vi "realtimecurrent.vi"() -> ()   [LabVIEW 2016]
uses:
  <vilib>/rvi/interface/nirviReadWriteControl/nirviReadWriteControl.xnode
  <vilib>/rvi/interface/nirviCloseFPGA/nirviCloseFPGA.xnode
  <vilib>/functionblocks/FB Core/FB Core.xnode
  <vilib>/rvi/interface/nirviOpenFPGA/nirviOpenFPGA.xnode
  <vilib>/userdefined/High Color/nirio_resource_hc.ctl
  NiFpgaLv.dll
  <vilib>/Utility/error.llb/Error Cluster From Error Code.vi
  <vilib>/rvi/errors/niLvFpgaAdjustHostInterfaceError.vi
  fpga/InjFPGA.vi
  <vilib>/functionblocks/Control/PID/PID.vi
  <vilib>/functionblocks/NI_FunctionBlock Libraries.lvlib
  FPGA Bitfiles/Controlsoftware2_FPGATarget_InjFPGA_-aTnSXeY2bA.lvbitx
  <vilib>/FPGAPlugInAG/cRIO-9074/niLvFpga_Open_cRIO-9074.vi
  <vilib>/FPGAPlugInAG/cRIO-9074/niLvFpga_Close_cRIO-9074.vi
panel:
  in  "x":dbl
  out "error out 6":errorcluster
  in  "Tab Control":enum32{"Controls", "Junk"}(tab)
  out "number":dbl=0.37297399999999997
  out "Stable 1":dbl=0.35939
  out "Rare":dbl=0.372956
  out "Light off Rare Light on Stable":bool
  out "Ion gauge Cluster 1":T1
  out "Waveform Chart":dbl(graph)=0.37297399999999997
  out "X-I":fxp<+/-,26,5>=1.2895498275756836 format="%.3g"
  out "X- V":fxp<+/-,26,5>=5.3390727043151855 format="%.3g"
  out "X+ I":fxp<+/-,26,5>=1.1065306663513184 format="%.3g"
  out "X+ V":fxp<+/-,26,5>=4.63661527633667 format="%.3g"
  out "Cryo pump":T2
  out "Stable field 2":dbl=0.3453
  in  "stop":bool
  out "Y+ V":fxp<+/-,26,5>=4.3806233406066895 format="%.3g"
  out "Y+I":fxp<+/-,26,5>=1.0684714317321777 format="%.3g"
  out "Y-V":fxp<+/-,26,5>=5.595516681671143 format="%.3g"
  out "Y-I":fxp<+/-,26,5>=1.365699291229248 format="%.3g"
  out "Pre-acc V":fxp<+/-,26,5>=8.250757694244385 format="%.3g"
  out "Preacc I":fxp<+/-,26,5>=2.544708251953125 format="%.3g"
  out "Einzel V":fxp<+/-,26,5>=7.414332389831543 format="%.3g"
  out "Einzel I":fxp<+/-,26,5>=1.6784825325012207 format="%.3g"
  out "Pre-acc":dbl=8.274062727880011
  out "Inj Einzel":dbl=7.43540107394125
  out "X Steerer +":dbl=4.646031981008041
  out "X Steerer -":dbl=5.353968018991959
  out "Y Steerer +":dbl=4.388287596043864
  out "Y Steerer -":dbl=5.611712403956136
  in  "proportional gain (Kc) 3":dbl=10.0
  out "inj image ap read":bool
  out "inj image cup read":bool=TRUE
  out "inj cup set value":bool=TRUE
  out "inj obj apt set value":bool
  out "reset 2":bool
  out "error out 3":errorcluster
  in  "error in":errorcluster
  out "error out 4":errorcluster={"status"=FALSE, "code"=-1950679034, "source"="Shared Variable in realtimecurrent.vi<APPEND>\nThis error or warning occurred while reading the following Shared Variable:\n\\\\inj-image-rio\\injfield_var\\oscillate\n\\\\192.168.1.105\\injfield_var\\oscillate"}
  out "unsigned byte array":u8[](array[numeric])=[87, 65, 32, 50, 49, 56, 54, 49, 56, 13]
  out "proportional gain (Kc)":dbl=1.0
  in  "integral time (Ti, min)":dbl=0.0005
  in  "derivative time (Td, min)":dbl=0.0005
  in  "auto? (T)":bool=TRUE
  out "stable1 or stable 2":bool=TRUE
  out "proportional gain (Kc) 2":dbl=2.0
  out "Convectron 2":u8[](array[numeric])
  out "Ion gauge 2":u8[](array[numeric])
  out "Convectron 1":u8[](array[numeric])
  out "Ion gauge 1":u8[](array[numeric])
  in  "Cryo pump 2":T3
  out "string":string="ff -0.372974T\n\r"
  out "error out 2":errorcluster
  out "error out 5":errorcluster
  out "error out":errorcluster
  out "substring before match":string="ff -0.372974"
  out "after substring":string="-0.372974"
  out "Array":u8[](array[numeric])=[102, 102, 32, 45, 48, 46, 51, 55, 50, 57, 55, 52, 84, 10, 13]
  out "Numeric":i32=1540
  out "concatenated string":string="WA 218618\r"
  in  "Ion gauge cluster control":T1
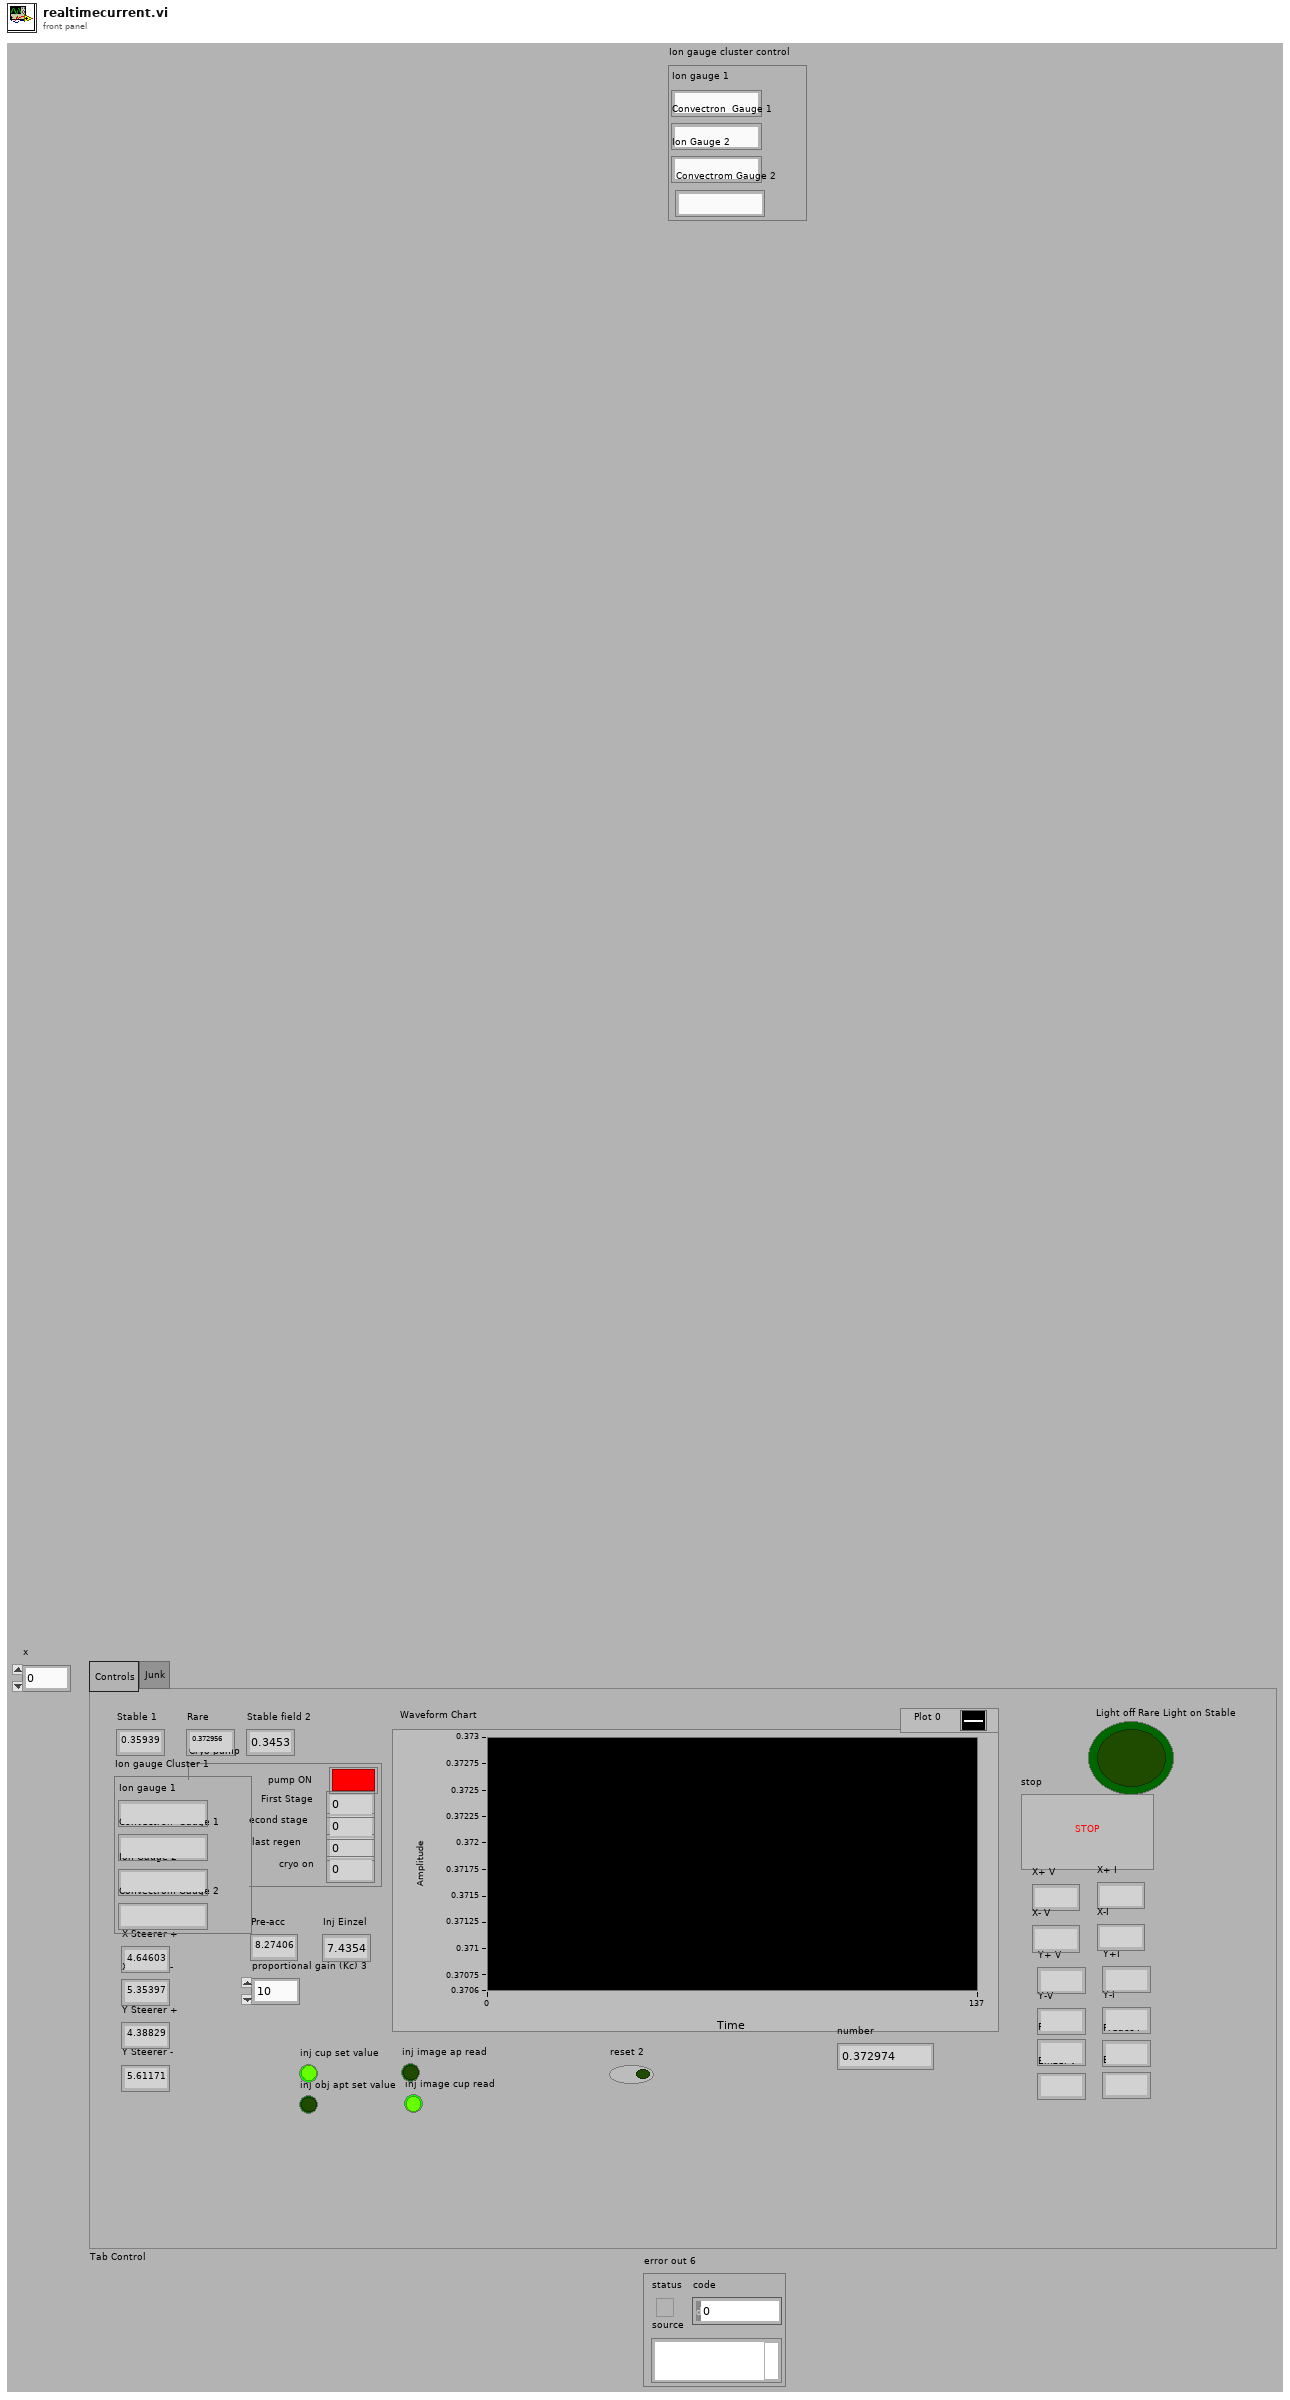
[diagram p1: front panel]
types:
  T1 = cluster{"Ion gauge 1":string, "Convectron  Gauge 1 ":string, "Ion Gauge 2":string, "Convectrom Gauge 2":string}
  T2 = cluster{"First Stage":dbl, "Second stage":dbl, "Hours since last regen":dbl, "pump ON":bool, "cryo on":dbl}
  T3 = cluster{"First Stage":dbl, "Second stage":dbl, "Hours since last regen":dbl, "Pump ON":bool, "Time on":dbl}
  T4 = typedef "nirio_resource_hc.ctl" = tag
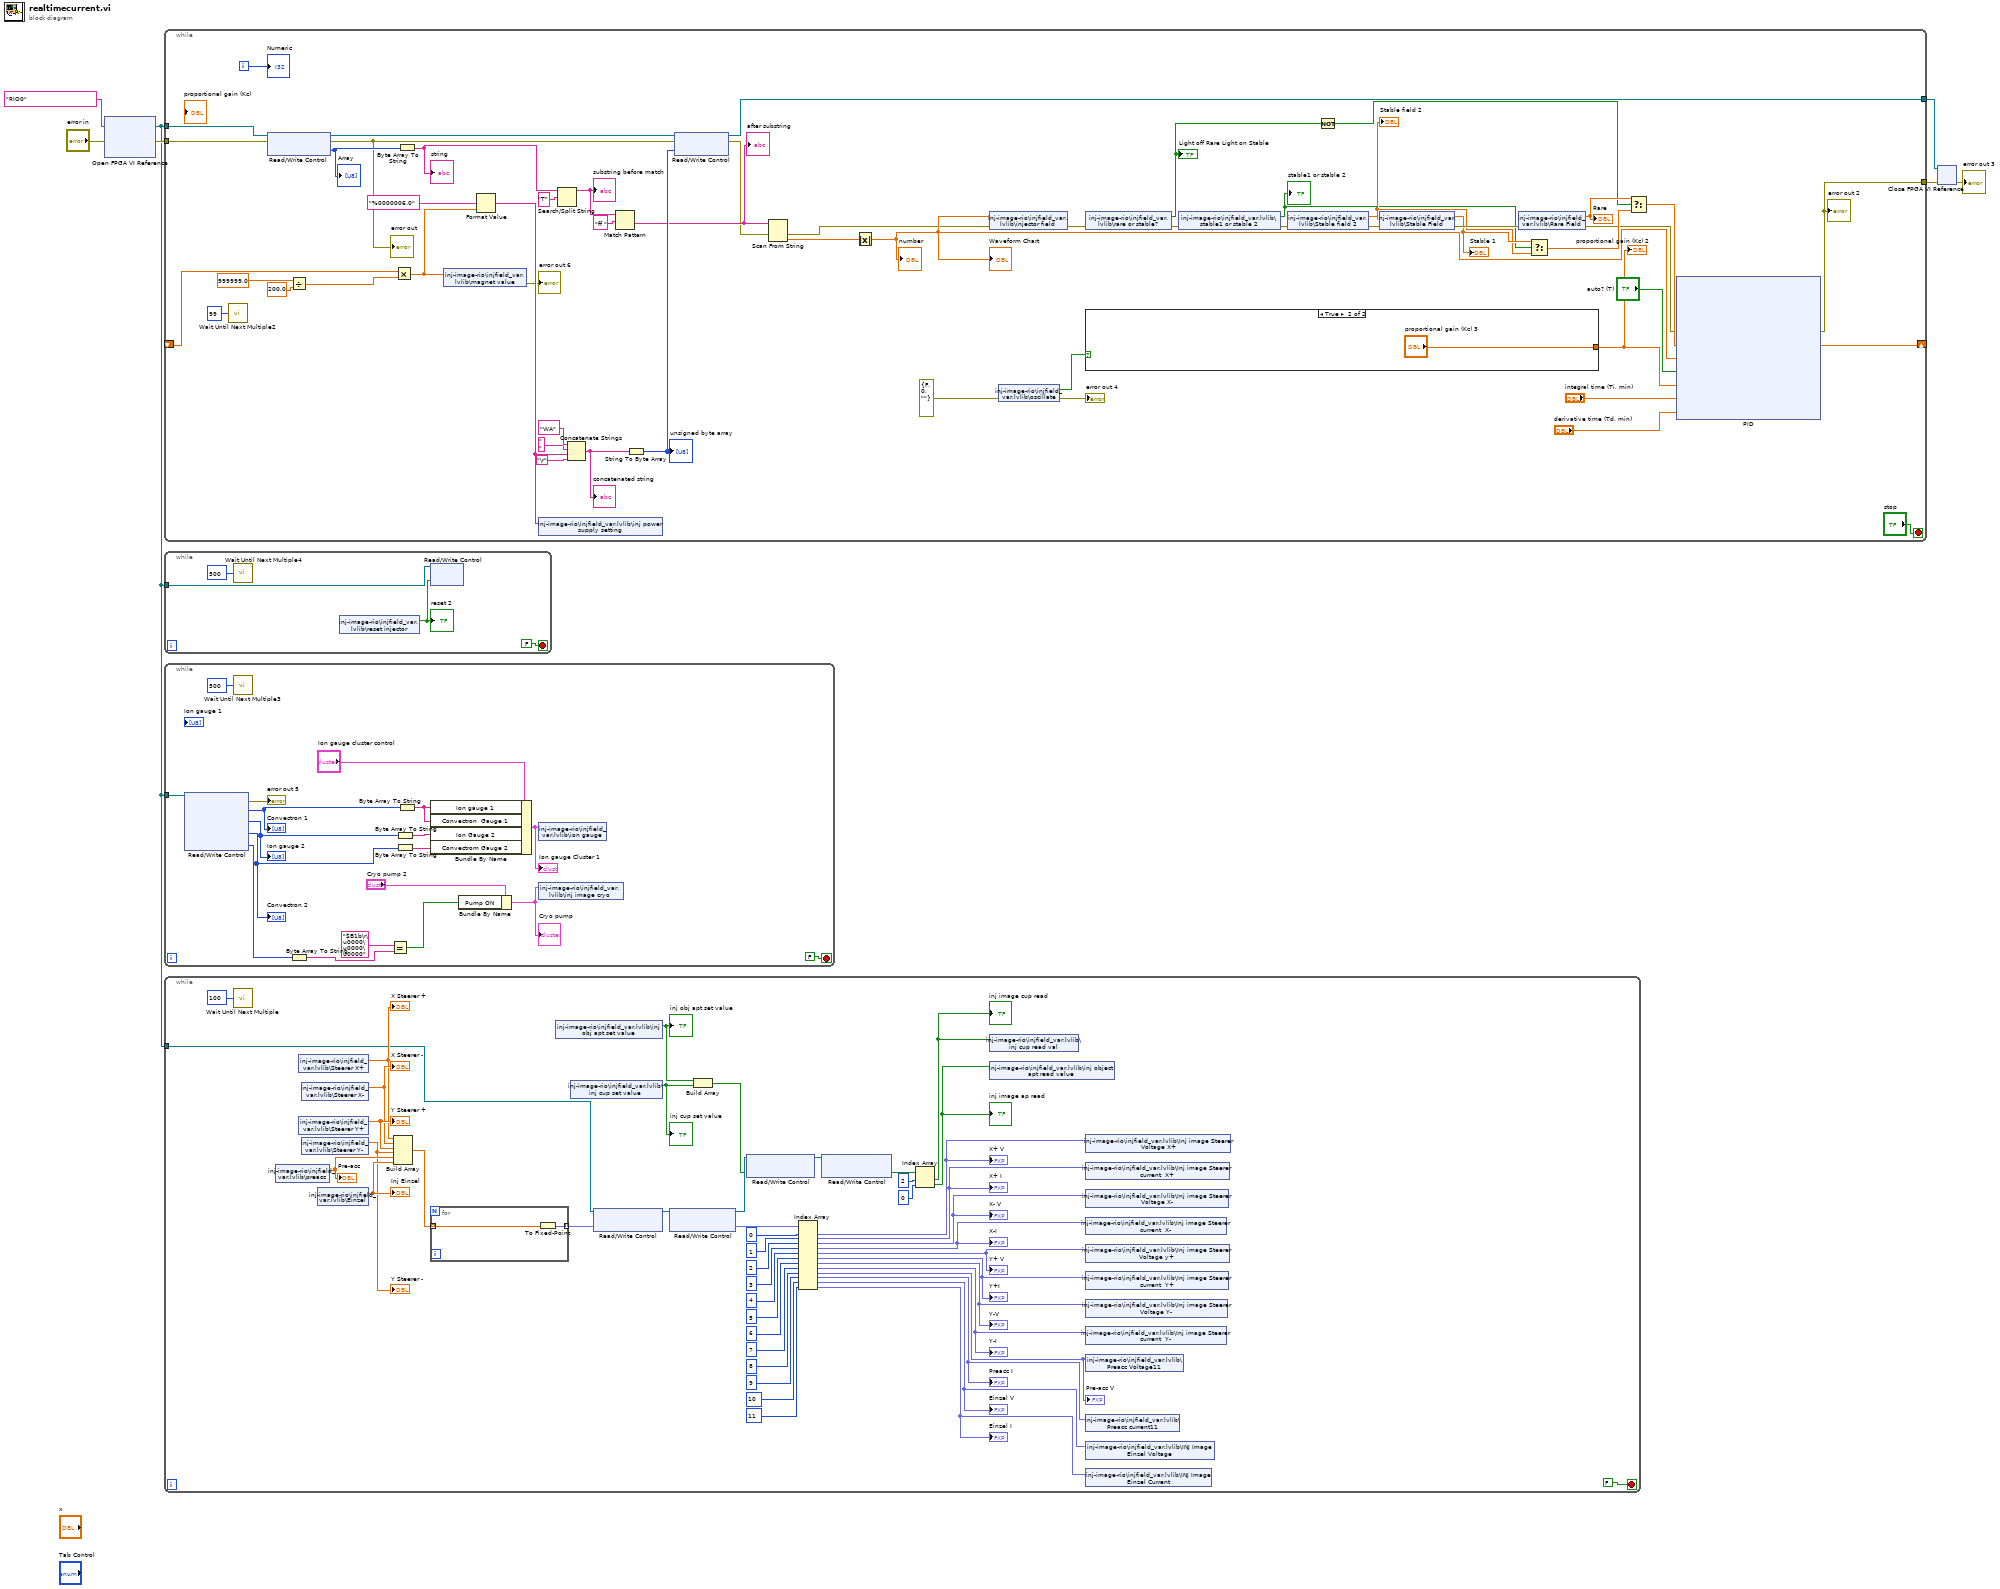
[diagram p0: block diagram]
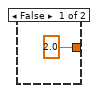
[diagram p2: hidden frame]
diagram:
  n1 = xnode "Open FPGA VI Reference"("error in"="error in", "resource name"=T4 "RIO0") -> ("FPGA VI Reference Out"=w1:refnum<k20>, "error out"=w3:errorcluster)
  n2 = while {
    tunnel: w1 -> [w8]
    tunnel: w3 -> [w61]
    tunnel: [w48] -> w7
    shift-right: [w40] -> _
    shift-left: _ -> [w9]
    tunnel: [w14] -> w6
    i -> [w58]
    stop <- "stop" stop-if-true
    n3 = call "Wait Until Next Multiple2"("Count(mSec)"=u32 99) -> ()  [unwired: 1 out]
    n4 = xnode "Read/Write Control"("FPGA VI Reference In"=w8, "error in"=w61) -> ("FPGA VI Reference Out"=w50:refnum<k20>, "error out"=w49:errorcluster, "magnet field"=w59:u8[])
    "Array" <- w59
    "error out" <- w49
    n5 = Divide(x=999999.0, y=200.0) -> (x/y=w55:dbl)
    n6 = Multiply(x=w9, y=w55) -> (x*y=w11:dbl)
    n7 = Byte Array To String(unsigned byte array=w59) -> (string=w45:string)
    "string" <- w45
    n8 = shared-variable "inj-image-rio\\injfield_var.lvlib\\magnet value"(w11) -> (error out=→"error out 6":errorcluster)  [unwired: 1 in]
    n9 = Format Value(format string="%0000006.0", value (0)=w11) -> (output string=w12:string)  [unwired: 1 out]
    n10 = shared-variable "inj-image-rio\\injfield_var.lvlib\\inj power supply setting"(w12) -> ()  [unwired: 1 in, 1 out]
    n11 = Search/Split String(string=w45, search string/char (-)="T") -> (substring before match=w43:string)  [unwired: 3 out]
    "substring before match" <- w43
    n12 = Concatenate Strings("WA", " ", w12, "\r") -> (w51:string)
    "concatenated string" <- w51
    n13 = Match Pattern(string=w43, regular expression="ff ") -> (after substring=w41:string)  [unwired: 4 out]
    "after substring" <- w41
    n14 = String To Byte Array(string=w51) -> (unsigned byte array=w47:u8[])
    "unsigned byte array" <- w47
    n15 = xnode "Read/Write Control"("FPGA VI Reference In"=w50, "error in"=w49, "magnet ps"=w47) -> ("FPGA VI Reference Out"=w48:refnum<k20>, "error out"=w19:errorcluster)
    n16 = Scan From String(input string=w41, error in=w19) -> (error out=w18:errorcluster, output 1=w38:dbl)  [unwired: 2 in, 3 out]
    n17 = Absolute Value(x=w38) -> (abs(x)=w33:dbl)
    "number" <- w33
    "Waveform Chart" <- w33
    n18 = shared-variable "inj-image-rio\\injfield_var.lvlib\\injector field"(w33, error in=w18) -> (error out=w32:errorcluster)
    n19 = shared-variable "inj-image-rio\\injfield_var.lvlib\\oscillate"(error in=errorcluster {"status"=FALSE, "code"=0, "source"=""} ("error in (no error)")) -> (w20:bool, error out=→"error out 4":errorcluster)
    n20 = shared-variable "inj-image-rio\\injfield_var.lvlib\\rare or stable?"(error in=w32) -> (w29:bool, error out=w27:errorcluster)
    "Light off Rare Light on Stable" <- w29
    n21 = case shown="True" w20 {
      tunnel: [2.0 ("proportional gain (Kc) 2") "proportional gain (Kc) 3"] -> w36
      frame False {
      }
      frame True {
      }
    }
    "proportional gain (Kc) 2" <- w36
    n22 = shared-variable "inj-image-rio\\injfield_var.lvlib\\stable1 or stable 2"(error in=w27) -> (w22:bool, error out=w26:errorcluster)
    "stable1 or stable 2" <- w22
    n23 = shared-variable "inj-image-rio\\injfield_var.lvlib\\Stable field 2"(error in=w26) -> (w23:dbl, error out=w25:errorcluster)
    "Stable field 2" <- w23
    n24 = Not(x=w29) -> (.not. x?=w28:bool)
    n25 = shared-variable "inj-image-rio\\injfield_var.lvlib\\Stable Field"(error in=w25) -> (w24:dbl, error out=w30:errorcluster)
    "Stable 1" <- w24
    n26 = shared-variable "inj-image-rio\\injfield_var.lvlib\\Rare Field"(error in=w30) -> (w31:dbl, error out=w17:errorcluster)
    "Rare" <- w31
    n27 = Select(t=w24, s=w22, f=w23) -> (s? t:f=w21:dbl)
    n28 = Select(t=w31, s=w28, f=w21) -> (s? t:f=w34:dbl)
    n29 = xnode "PID"("error in"=w17, "setpoint"=w34, "process variable"=w33, "auto? (T)"="auto? (T)", "proportional gain (Kc)"=w36, "integral time (Ti, min)"="integral time (Ti, min)", "derivative time (Td, min)"="derivative time (Td, min)") -> ("error out"=w14:errorcluster, "output"=w40:dbl)
    "error out 2" <- w14
    "Numeric" <- w58
  }
  n30 = while {
    tunnel: w1 -> [w131]
    stop <- FALSE stop-if-true
    n31 = call "Wait Until Next Multiple4"("Count(mSec)"=u32 500) -> ()  [unwired: 1 out]
    n32 = shared-variable "inj-image-rio\\injfield_var.lvlib\\reset injector"() -> (w130:bool)  [unwired: 1 in, 1 out]
    "reset 2" <- w130
    n33 = xnode "Read/Write Control"("FPGA VI Reference In"=w131, "reset"=w130) -> ()  [unwired: 1 in, 2 out]
  }
  n34 = while {
    tunnel: w1 -> [w147]
    stop <- FALSE stop-if-true
    n35 = xnode "Read/Write Control"("FPGA VI Reference In"=w147) -> ("error out"=→"error out 5":errorcluster, "Convectron 3"=w146:u8[], "Convectron 4"=w145:u8[], "Ion gauge 4"=w135:u8[], "Pump On"=w139:u8[])  [unwired: 1 in, 1 out]
    "Convectron 1" <- w146
    "Ion gauge 2" <- w145
    "Convectron 2" <- w135
    n36 = call "Wait Until Next Multiple3"("Count(mSec)"=u32 500) -> ()  [unwired: 1 out]
    n37 = Byte Array To String(unsigned byte array=w139) -> (string=w141:string)
    n38 = Equal?(x="$B1b\r\u0000\u0000\u0000" ("string 2"), y=w141) -> (x = y?=w138:bool)
    n39 = Byte Array To String(unsigned byte array=w145) -> (string=w149:string)
    n40 = Byte Array To String(unsigned byte array=w135) -> (string=w148:string)
    n41 = Byte Array To String(unsigned byte array=w146) -> (string=w134:string)
    n42 = Bundle By Name(cluster="Ion gauge cluster control", "Ion gauge 1"=w134, "Convectron  Gauge 1"=w134, "Ion Gauge 2"=w149, "Convectrom Gauge 2"=w148) -> (w137:T1)
    "Ion gauge Cluster 1" <- w137
    n43 = Bundle By Name(cluster="Cryo pump 2", "Pump ON"=w138) -> (w136:T3)
    "Cryo pump" <- w136
    n44 = shared-variable "inj-image-rio\\injfield_var.lvlib\\ion gauge"(w137) -> ()  [unwired: 1 in, 1 out]
    n45 = shared-variable "inj-image-rio\\injfield_var.lvlib\\inj image cryo"(w136) -> ()  [unwired: 1 in, 1 out]
  }
  n46 = while {
    tunnel: w1 -> [w164]
    stop <- FALSE stop-if-true
    n47 = call "Wait Until Next Multiple"("Count(mSec)"=u32 100) -> ()  [unwired: 1 out]
    n48 = shared-variable "inj-image-rio\\injfield_var.lvlib\\preacc"() -> (w184:dbl)  [unwired: 1 in, 1 out]
    "Pre-acc" <- w184
    n49 = shared-variable "inj-image-rio\\injfield_var.lvlib\\Steerer X+"() -> (w179:dbl)  [unwired: 1 in, 1 out]
    "X Steerer +" <- w179
    n50 = shared-variable "inj-image-rio\\injfield_var.lvlib\\Steerer Y+"() -> (w181:dbl)  [unwired: 1 in, 1 out]
    "Y Steerer +" <- w181
    n51 = shared-variable "inj-image-rio\\injfield_var.lvlib\\Steerer X-"() -> (w180:dbl)  [unwired: 1 in, 1 out]
    "X Steerer -" <- w180
    n52 = shared-variable "inj-image-rio\\injfield_var.lvlib\\Steerer Y-"() -> (w182:dbl)  [unwired: 1 in, 1 out]
    "Y Steerer -" <- w182
    n53 = shared-variable "inj-image-rio\\injfield_var.lvlib\\Einzel"() -> (w183:dbl)  [unwired: 1 in, 1 out]
    "Inj Einzel" <- w183
    n54 = Build Array(w179, w180, w181, w182, w184, w183) -> (w162:dbl[])
    n55 = for {
      tunnel: [w200] -> w163 mode=indexing
      tunnel: w162 -> [w199] mode=indexing
      n56 = To Fixed-Point(number=w199) -> (fixed-point=w200:fxp<+/-,32,16>)  [unwired: 1 in]
    }
    n57 = shared-variable "inj-image-rio\\injfield_var.lvlib\\inj obj apt set value"() -> (w153:bool)  [unwired: 1 in, 1 out]
    "inj obj apt set value" <- w153
    n58 = shared-variable "inj-image-rio\\injfield_var.lvlib\\inj cup set value"() -> (w152:bool)  [unwired: 1 in, 1 out]
    "inj cup set value" <- w152
    n59 = xnode "Read/Write Control"("FPGA VI Reference In"=w164, "analog output"=w163) -> ("FPGA VI Reference Out"=w185:refnum<k20>)  [unwired: 1 in, 1 out]
    n60 = xnode "Read/Write Control"("FPGA VI Reference In"=w185) -> ("FPGA VI Reference Out"=w160:refnum<k20>, "Analog input"=w198:fxp<+/-,26,5>[])  [unwired: 1 in, 1 out]
    n61 = Build Array(w153, w152) -> (w159:bool[])
    n62 = xnode "Read/Write Control"("FPGA VI Reference In"=w160, "cup set values"=w159) -> ("FPGA VI Reference Out"=w161:refnum<k20>)  [unwired: 1 in, 1 out]
    n63 = Index Array(array=w198, index #1=0 ("index"), index #2=1 ("index"), index #3=2 ("index"), index #4=3 ("index"), index #5=4 ("index"), index #6=5 ("index"), index #7=6 ("index"), index #8=7 ("index"), index #9=8 ("index"), index #10=9 ("index"), index #11=10 ("index"), index #12=11 ("index")) -> (element #1=w171:fxp<+/-,26,5>, element #2=w167:fxp<+/-,26,5>, element #3=w172:fxp<+/-,26,5>, element #4=w168:fxp<+/-,26,5>, element #5=w173:fxp<+/-,26,5>, element #6=w169:fxp<+/-,26,5>, element #7=w174:fxp<+/-,26,5>, element #8=w170:fxp<+/-,26,5>, element #9=w175:fxp<+/-,26,5>, element #10=w176:fxp<+/-,26,5>, element #11=w166:fxp<+/-,26,5>, element #12=w165:fxp<+/-,26,5>)
    "Y+ V" <- w173
    "Y+I" <- w169
    "Y-V" <- w174
    "Y-I" <- w170
    "Pre-acc V" <- w175
    "Preacc I" <- w176
    "Einzel V" <- w166
    "Einzel I" <- w165
    "X+ V" <- w171
    "X+ I" <- w167
    "X- V" <- w172
    "X-I" <- w168
    n64 = xnode "Read/Write Control"("FPGA VI Reference In"=w161) -> ("cup readbacks"=w158:bool[])  [unwired: 1 in, 2 out]
    n65 = Index Array(array=w158, index #1=2 ("index"), index #2=0 ("index")) -> (element #1=w155:bool, element #2=w154:bool)
    "inj image ap read" <- w154
    "inj image cup read" <- w155
    n66 = shared-variable "inj-image-rio\\injfield_var.lvlib\\inj cup read val"(w155) -> ()  [unwired: 1 in, 1 out]
    n67 = shared-variable "inj-image-rio\\injfield_var.lvlib\\inj object apt read value"(w154) -> ()  [unwired: 1 in, 1 out]
    n68 = shared-variable "inj-image-rio\\injfield_var.lvlib\\Inj image Steerer Voltage X+"(w171) -> ()  [unwired: 1 in, 1 out]
    n69 = shared-variable "inj-image-rio\\injfield_var.lvlib\\Inj image Steerer current  X+"(w167) -> ()  [unwired: 1 in, 1 out]
    n70 = shared-variable "inj-image-rio\\injfield_var.lvlib\\Inj image Steerer Voltage X-"(w172) -> ()  [unwired: 1 in, 1 out]
    n71 = shared-variable "inj-image-rio\\injfield_var.lvlib\\Inj image Steerer current  X-"(w168) -> ()  [unwired: 1 in, 1 out]
    n72 = shared-variable "inj-image-rio\\injfield_var.lvlib\\Inj image Steerer Voltage y+"(w173) -> ()  [unwired: 1 in, 1 out]
    n73 = shared-variable "inj-image-rio\\injfield_var.lvlib\\Inj image Steerer current  Y+"(w169) -> ()  [unwired: 1 in, 1 out]
    n74 = shared-variable "inj-image-rio\\injfield_var.lvlib\\Inj image Steerer Voltage Y-"(w174) -> ()  [unwired: 1 in, 1 out]
    n75 = shared-variable "inj-image-rio\\injfield_var.lvlib\\Inj image Steerer current  Y-"(w170) -> ()  [unwired: 1 in, 1 out]
    n76 = shared-variable "inj-image-rio\\injfield_var.lvlib\\Preacc Voltage11"(w175) -> ()  [unwired: 1 in, 1 out]
    n77 = shared-variable "inj-image-rio\\injfield_var.lvlib\\Preacc current11"(w176) -> ()  [unwired: 1 in, 1 out]
    n78 = shared-variable "inj-image-rio\\injfield_var.lvlib\\INJ Image Einzel Voltage"(w166) -> ()  [unwired: 1 in, 1 out]
    n79 = shared-variable "inj-image-rio\\injfield_var.lvlib\\INJ Image Einzel Current"(w165) -> ()  [unwired: 1 in, 1 out]
  }
  n80 = xnode "Close FPGA VI Reference"("FPGA VI Reference In"=w7, "error in"=w6) -> ("error out"=→"error out 3":errorcluster)
